vi "Read Value (variant).vi"(8 "error in (no error)":errorcluster, 11 "Double D Element in":refnum<class "Double D Element.lvclass">) -> (0 "error out":errorcluster, 2 "Variant":variant, 3 "Double D Element out":refnum<class "Double D Element.lvclass">)   [LabVIEW 2018, in "D Datagrid Library.lvlib" / "Double D Element.lvclass"]
uses:
  Double D Element.lvclass
  Double D Element.lvclass/Double D Element.ctl
  Read Value.vi
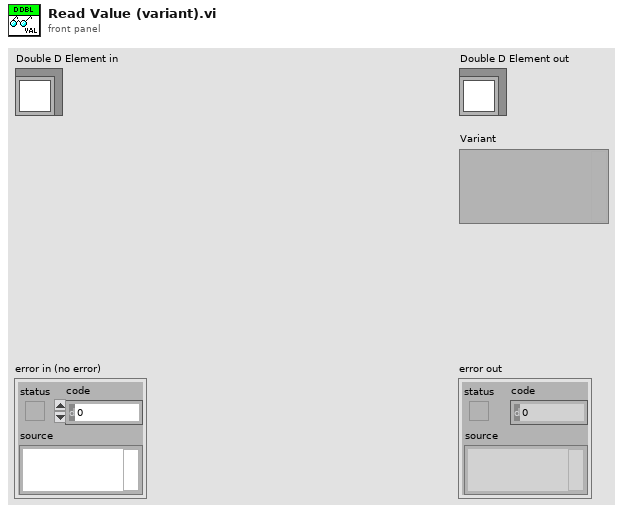
[diagram p1: front panel]
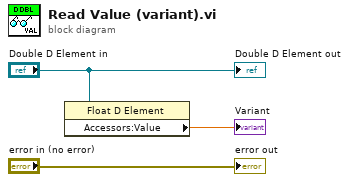
[diagram p0: block diagram]
diagram:
  n1 = property class="Float D Element"(reference="Double D Element in") -> ("Accessors:Value"=→"Variant":dbl)  [unwired: 1 in, 2 out]
  "error out" <- "error in (no error)"
  "Double D Element out" <- "Double D Element in"
